vi "Advance Edge find result.vi"(6 "Scalling Value":string[][](array[string]), 8 "error in (no error)":errorcluster, 9 "Vision Tool":string, 10 "Image":T1(plugin-control), 11 "List box Value":string[][](array[string])) -> (0 "error out":errorcluster, 1 "ADVANCED EDGE PROCESSING Result":T2(array[cluster]), 3 "Image":T1(plugin-control))   [LabVIEW 2020]
uses:
  <vilib>/vision/Measure.llb/Edge Options.ctl
  <vilib>/vision/Measure.llb/Edge Polarity.ctl
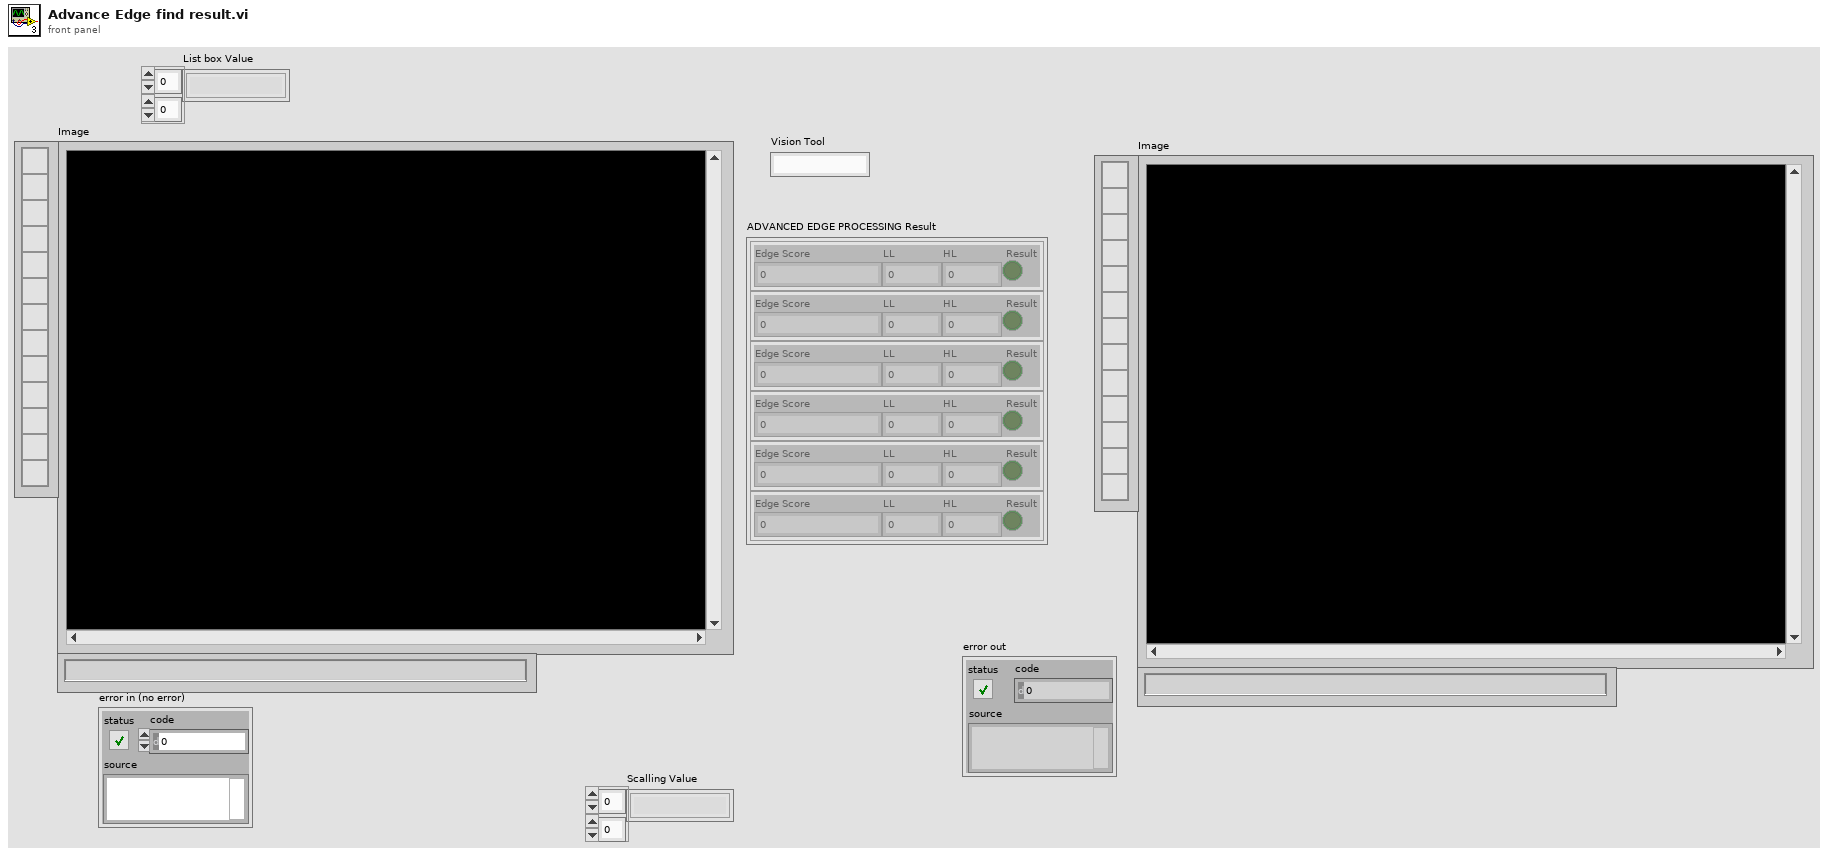
[diagram p1: front panel]
types:
  T1 = typedef "IMAQ Image.ctl" = refnum<image>
  T2 = cluster{"Edge Score":dbl, "LL":dbl, "HL":dbl, " Result":bool}[]
  T3 = enum32{"Zero Order", "Bilinear", "Quadratic", "Cubic", "Bilinear Fixed"}
  T4 = typedef "Edge Options.ctl" = cluster{"Edge Polarity":T5, "Kernel Size":u32, "Width":u32, "Minimum Edge Strength":sgl, "Interpolation Type":enum32{"Zero Order", "Bilinear", "Quadratic", "Cubic", "Bilinear Fixed"}, "Data Processing Method":enum32{"Average", "Median"}}
  T5 = typedef "Edge Polarity.ctl" = u32
  T6 = enum16{"Get First Edge", "Get First + Last Edge", "Get All Edges", "Get Best Edge"}
  T7 = cluster{"Global Rectangle":i32[], "Contours":cluster{"Contour Type":u32, "ROI Type":u32, "Points":i32[]}[]}
  T8 = enum16{"Subtract Fixturing Values ", "Add Fixturing Values"}
  T9 = cluster{i32[], cluster{"Contour Type":u32, "Contour Type":i32, i32[]}[]}
  T10 = typedef "Edge New.ctl" = cluster{"Location (Pixel)":cluster{"X":sgl, "Y":sgl}, "Location (Real-World)":cluster{"X":sgl, "Y":sgl}, "Distance (Pixel)":dbl, "Distance (Real-World)":dbl, "Strength":dbl, "Noise":dbl, "Rising?":bool}
  T11 = cluster{"Lower Limit":dbl, "Higher Limit":dbl, "Length":dbl, "Result":bool}[]
  T12 = cluster{"Edge Score":dbl, "LL":dbl, "HL":dbl, " Result":bool}
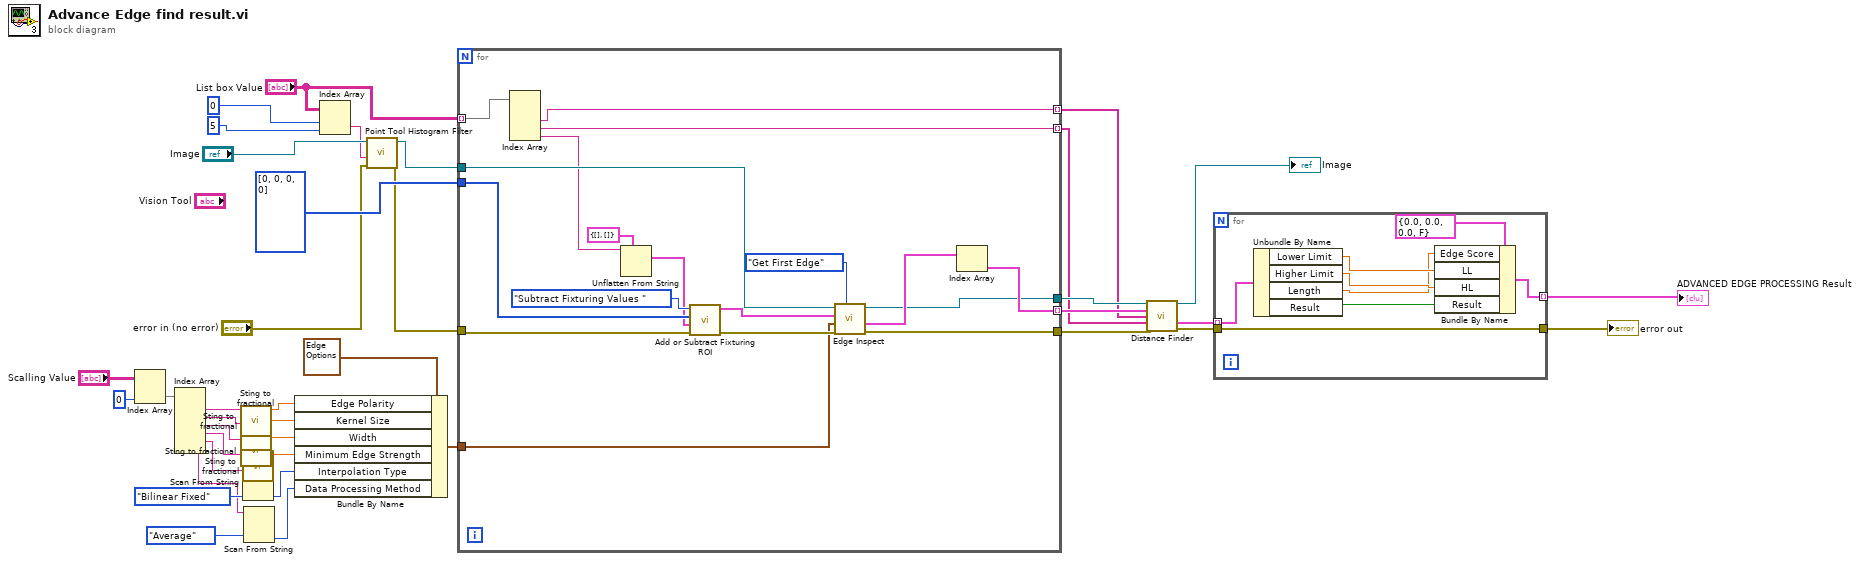
[diagram p0: block diagram]
diagram:
  n1 = Index Array(array="Scalling Value", index (col)=0 ("disabled index (col)")) -> (element=w16:string[])  [unwired: 1 in]
  n2 = Index Array(array=w16) -> (element #1=w15:string, element #2=w14:string, element #3=w13:string, element #4=w9:string, element #5=w6:string, element #6=w4:string)  [unwired: 6 in]
  n3 = call "Sting to fractional.vi"("String"=w15) -> ("Numeric"=w12:dbl)  [unwired: 10 in]
  n4 = call "Sting to fractional.vi"("String"=w14) -> ("Numeric"=w11:dbl)  [unwired: 10 in]
  n5 = call "Sting to fractional.vi"("String"=w13) -> ("Numeric"=w10:dbl)  [unwired: 10 in]
  n6 = call "Sting to fractional.vi"("String"=w9) -> ("Numeric"=w8:dbl)  [unwired: 10 in]
  n7 = Scan From String(input string=w6, default 1=T3."Bilinear Fixed" ("Interpolation Type")) -> (output 1=w5:T3)  [unwired: 3 in, 3 out]
  n8 = Scan From String(input string=w4, default 1=enum32{"Average", "Median"}."Average" ("Data Processing Method")) -> (output 1=w2:enum32{"Average", "Median"})  [unwired: 3 in, 3 out]
  n9 = Bundle By Name(cluster=T4 {"Edge Polarity"=0, "Kernel Size"=3, "Width"=7, "Minimum Edge Strength"=10.0, "Interpolation Type"=enum."Bilinear Fixed", "Data Processing Method"=enum."Average"} ("Edge Options"), "Edge Polarity"=w12, "Kernel Size"=w11, "Width"=w10, "Minimum Edge Strength"=w8, "Interpolation Type"=w5, "Data Processing Method"=w2) -> (w1:T4)
  n10 = Index Array(array="List box Value", index (row)=0, index (col)=5 ("disabled index (col)")) -> (element=w22:string)
  n11 = call "Point Tool Histogram Filter.vi"("error in"="error in (no error)", "Combo Box"=w22, "Image in"="Image") -> ("error out"=w20:errorcluster, "Image out"=w26:T1)  [unwired: 7 in]
  n12 = for {
    tunnel: i32[] [0, 0, 0, 0] ("Fixturing ROI") -> [w55]
    tunnel: w20 -> [w51]
    tunnel: w26 -> [w50]
    tunnel: "List box Value" -> [w48] mode=indexing
    tunnel: [w45] -> w37 mode=indexing
    tunnel: [w44] -> w36
    tunnel: [w43] -> w35
    tunnel: [w42] -> w34 mode=indexing
    tunnel: [w40] -> w33 mode=indexing
    tunnel: w1 -> [w39]
    n13 = Index Array(array=w48) -> (element #2=w42:string, element #3=w40:string, element #4=w47:string)  [unwired: 4 in, 1 out]
    n14 = Unflatten From String(type=T7 {"Global Rectangle"=[], "Contours"=[]} ("ROI"), binary string=w47) -> (value=w41:T7)  [unwired: 3 in, 2 out]
    n15 = call "Add or Subtract Fixturing ROI.vi"("error control"=w51, "ROI in"=w41, "Fixturing ROI"=w55, "Enum"=T8."Subtract Fixturing Values ") -> ("error indicator"=w52:errorcluster, "ROI out"=w49:T9)  [unwired: 6 in]
    n16 = call "Edge Inspect.vi"("Process"=T6."Get First Edge", "error in (no error)"=w52, "Edge Options"=w39, "ROI Descriptor"=w49, "Main_RGB"=w50) -> ("error out"=w43:errorcluster, "Edge Information"=w46:T10[], "Image"=w44:T1)  [unwired: 3 in, 1 out]
    n17 = Index Array(array=w46) -> (element=w45:T10)  [unwired: 1 in]
  }
  n18 = call "Distance Finder.vi"("Grey in"=w36, "Array"=w37, "LL"=w34, "HL"=w33, "error in (no error)"=w35) -> ("RGB out"=→"Image":T1, "Analysis"=w31:T11, "error out"=w29:errorcluster)  [unwired: 8 in]
  n19 = for {
    tunnel: w31 -> [w63] mode=indexing
    tunnel: [w58] -> w30 mode=indexing
    tunnel: w29 -> [w57]
    tunnel: [w57] -> w28
    n20 = Unbundle By Name(w63) -> ("Lower Limit"=w62:dbl, "Higher Limit"=w61:dbl, "Length"=w60:dbl, "Result"=w59:bool)
    n21 = Bundle By Name(cluster=T12 {"Edge Score"=0.0, "LL"=0.0, "HL"=0.0, " Result"=FALSE} ("Pattern Single Result"), "Edge Score"=w60, "LL"=w62, "HL"=w61, "Result"=w59) -> (w58:T12)
  }
  "error out" <- w28
  "ADVANCED EDGE PROCESSING Result" <- w30
